vi "Convert to DAC Units.vi"(0 "Offset":dbl, 1 "Slope":dbl, 5 "Mass":dbl, 7 "Ch#":u8, 9 "coerced(x)":dbl, 11 "error in (no error)":errorcluster, 12 "s? t:f":dbl, 13 "Units":bool) -> (4 "OP 1":dbl, 6 "OP 2":dbl, 8 "OP 3":dbl, 10 "OP 4":dbl, 15 "error out":errorcluster)   [LabVIEW 2018]
uses:
  Type Defs/Global Action.ctl
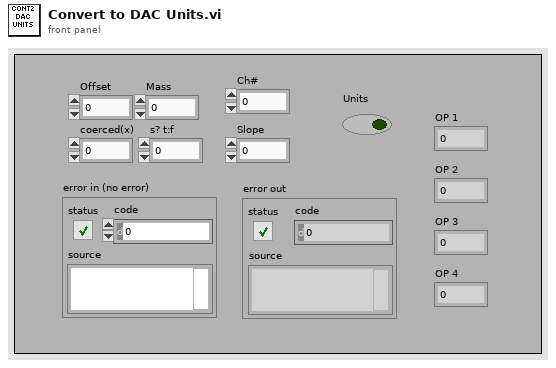
[diagram p1: front panel]
types:
  T1 = typedef "Global Action.ctl" = enum16{"Write", "Read"}
  T2 = typedef "Global Parameters.ctl" = cluster{"Calibrations":cluster{"Q1 +ve":dbl[][], "Q2 +ve":dbl[][], "Q1 -ve":dbl[][], "Q2 -ve":dbl[][]}, "Resolution Q1":cluster{"High +ve":dbl[][], "Med +ve":dbl[][], "Low +ve":dbl[][], "High -ve":dbl[][], "Med -ve":dbl[][], "Low -ve":dbl[][]}, "Resolution Q2":cluster{"High +ve":dbl[][], "Med +ve":dbl[][], "Loe +ve":dbl[][], "High -ve":dbl[][], "Med -ve":dbl[][], "Low -ve":dbl[][]}, "MR Parameters":T3, "Mass":dbl[][], "Dwell":dbl[][], "Steps":i32[][], "Method Refnum":refnum<vi>}
  T3 = typedef "MR Parameters.ctl" = cluster{"Name":string, "Ch#":u8, "StartV":dbl, "StopV":dbl, "StepV":dbl, "Index":u8}
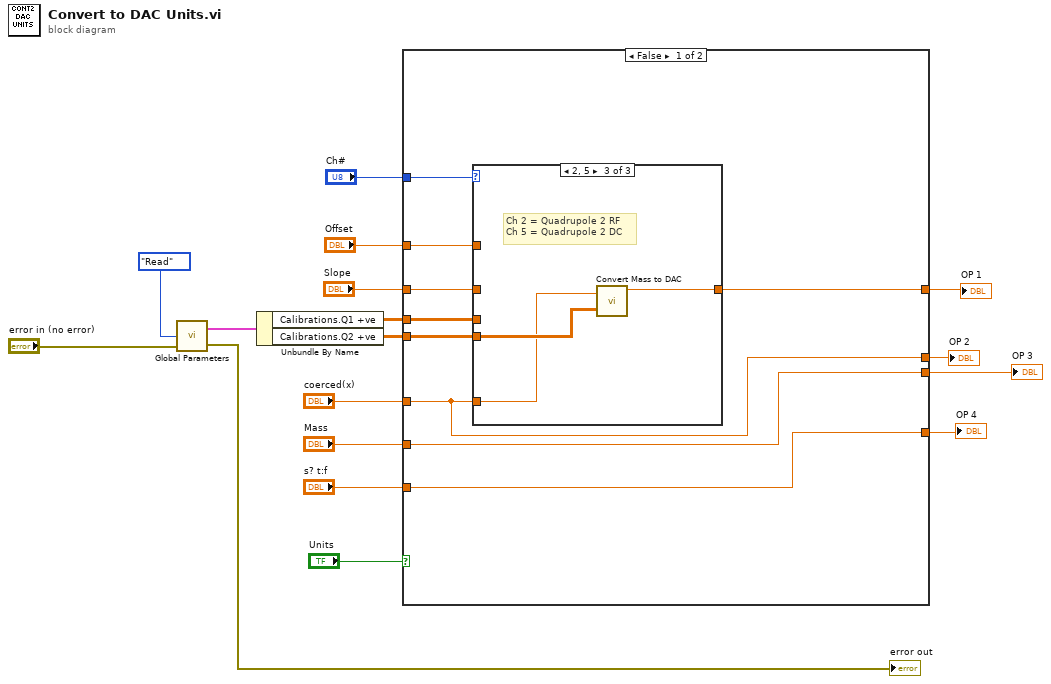
[diagram p0: block diagram]
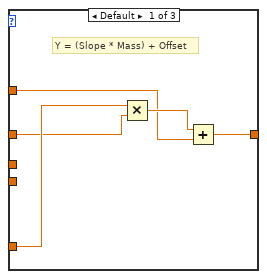
[diagram p2: hidden frame]
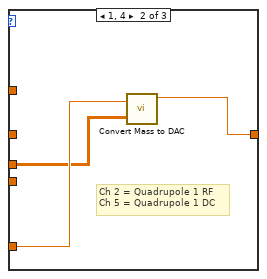
[diagram p3: hidden frame]
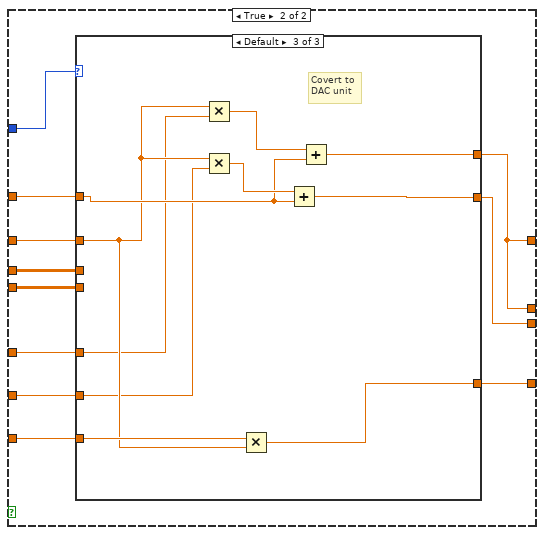
[diagram p4: hidden frame]
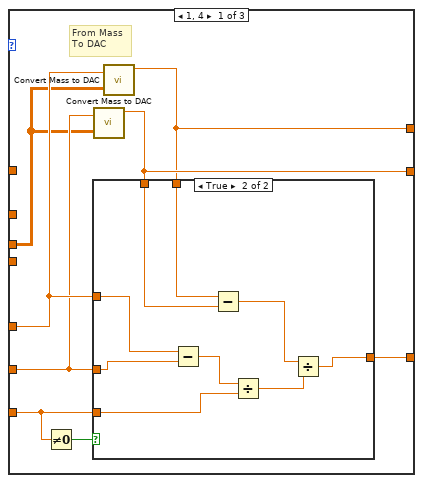
[diagram p5: hidden frame]
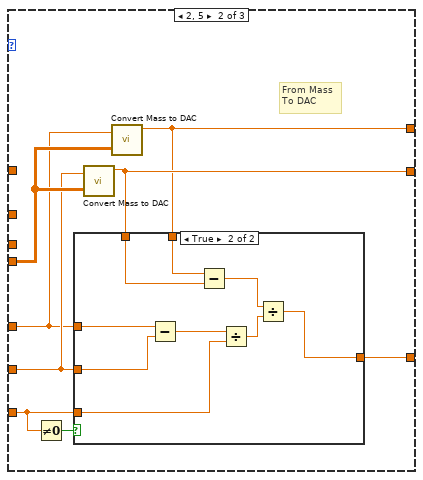
[diagram p7: hidden frame]
diagram:
  n1 = call "Global Parameters.vi"("Error In"="error in (no error)", "Action"=Global_Action."Read") -> ("Error Out"=→"error out":errorcluster, "Parameters Out"=w16:T2)  [unwired: 1 in]
  n2 = Unbundle By Name(w16) -> ("Calibrations.Q1 +ve"=w15:dbl[][], "Calibrations.Q2 +ve"=w14:dbl[][])
  n3 = case shown="False" "Units" {
    tunnel: [w20 w38] -> w2
    tunnel: [w19 w48] -> w3
    tunnel: [w18 w47] -> w4
    tunnel: "Ch#" -> [w26 w46]
    tunnel: w15 -> [w22 w40]
    tunnel: w14 -> [w21 w39]
    tunnel: "Offset" -> [w24 w43]
    tunnel: "Slope" -> [w25 w44]
    tunnel: "coerced(x)" -> [w20 w42]
    tunnel: "Mass" -> [w19 w41]
    tunnel: "s? t:f" -> [w18 w45]
    tunnel: [w23 w38] -> w1
    frame False {
      n4 = case shown="2, 5" w26 {
        tunnel: [w30 w32 w37] -> w23
        tunnel: w20 -> [w29 w34 w35]
        tunnel: w25 -> [w28 _ _]
        tunnel: w24 -> [w27 _ _]
        tunnel: w22 -> [_ w33 _]
        tunnel: w21 -> [_ _ w36]
        frame Default {
          # "Y = (Slope * Mass) + Offset"
          n5 = Multiply(x=w29, y=w28) -> (x*y=w31:dbl)
          n6 = Add(x=w31, y=w27) -> (x+y=w30:dbl)
        }
        frame 1, 4 {
          # "Ch 2 = Quadrupole 1 RF\nCh 5 = Quadrupole 1 DC"
          n7 = call "Convert Mass to DAC.vi"("Mass"=w34, "Calibration Table"=w33) -> ("DAC Value"=w32:dbl)  [unwired: 3 out]
        }
        frame 2, 5 {
          # "Ch 2 = Quadrupole 2 RF\nCh 5 = Quadrupole 2 DC"
          n8 = call "Convert Mass to DAC.vi"("Mass"=w35, "Calibration Table"=w36) -> ("DAC Value"=w37:dbl)  [unwired: 3 out]
        }
      }
    }
    frame True {
      n9 = case shown="Default" w46 {
        tunnel: [w50 w71 w93] -> w38
        tunnel: [w54 w72 w91] -> w48
        tunnel: [w56 w74 w90] -> w47
        tunnel: w45 -> [w49 w69 w89]
        tunnel: w44 -> [_ _ w87]
        tunnel: w43 -> [_ _ w88]
        tunnel: w42 -> [w53 w67 w86]
        tunnel: w41 -> [w52 w68 w85]
        tunnel: w40 -> [w51 _ _]
        tunnel: w39 -> [_ w70 _]
        frame 1, 4 {
          # "From Mass\nTo DAC"
          n10 = Not Equal To 0?(x=w49) -> (x != 0?=w55:bool)
          n11 = call "Convert Mass to DAC.vi"("Mass"=w52, "Calibration Table"=w51) -> ("DAC Value"=w54:dbl)  [unwired: 3 out]
          n12 = call "Convert Mass to DAC.vi"("Mass"=w53, "Calibration Table"=w51) -> ("DAC Value"=w50:dbl)  [unwired: 3 out]
          n13 = case shown="True" w55 {
            tunnel: [w57 w63] -> w56
            tunnel: w54 -> [_ w59]
            tunnel: w53 -> [_ w62]
            tunnel: w52 -> [_ w61]
            tunnel: w50 -> [_ w60]
            tunnel: w49 -> [w57 w58]
            frame False {
            }
            frame True {
              n14 = Subtract(x=w62, y=w61) -> (x-y=w64:dbl)
              n15 = Subtract(x=w60, y=w59) -> (x-y=w65:dbl)
              n16 = Divide(x=w64, y=w58) -> (x/y=w66:dbl)
              n17 = Divide(x=w65, y=w66) -> (x/y=w63:dbl)
            }
          }
        }
        frame 2, 5 {
          # "From Mass\nTo DAC"
          n18 = Not Equal To 0?(x=w69) -> (x != 0?=w73:bool)
          n19 = call "Convert Mass to DAC.vi"("Mass"=w68, "Calibration Table"=w70) -> ("DAC Value"=w72:dbl)  [unwired: 3 out]
          n20 = call "Convert Mass to DAC.vi"("Mass"=w67, "Calibration Table"=w70) -> ("DAC Value"=w71:dbl)  [unwired: 3 out]
          n21 = case shown="True" w73 {
            tunnel: w71 -> [_ w81]
            tunnel: w72 -> [_ w80]
            tunnel: [w75 w79] -> w74
            tunnel: w69 -> [w75 w78]
            tunnel: w68 -> [_ w77]
            tunnel: w67 -> [_ w76]
            frame False {
            }
            frame True {
              n22 = Subtract(x=w76, y=w77) -> (x-y=w82:dbl)
              n23 = Subtract(x=w81, y=w80) -> (x-y=w83:dbl)
              n24 = Divide(x=w82, y=w78) -> (x/y=w84:dbl)
              n25 = Divide(x=w83, y=w84) -> (x/y=w79:dbl)
            }
          }
        }
        frame Default {
          # "Covert to\nDAC unit"
          n26 = Multiply(x=w87, y=w86) -> (x*y=w94:dbl)
          n27 = Multiply(x=w87, y=w85) -> (x*y=w92:dbl)
          n28 = Multiply(x=w89, y=w87) -> (x*y=w90:dbl)
          n29 = Add(x=w92, y=w88) -> (x+y=w91:dbl)
          n30 = Add(x=w94, y=w88) -> (x+y=w93:dbl)
        }
      }
    }
  }
  "OP 4" <- w4
  "OP 3" <- w3
  "OP 2" <- w2
  "OP 1" <- w1
